vi "UI Loop - RT Target Monitoring.vi"(11 "Message Queue Reference":refnum<queue> caption="消息队列引用") -> ()   [LabVIEW 2015]
uses:
  Support VIs/Message Queue/Message Cluster.ctl
  Globals/Global - All UI Loop Stop.vi
  Support VIs/Message Queue/Message Queue.lvlib
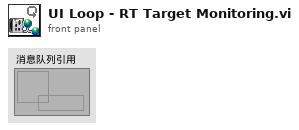
[diagram p1: front panel]
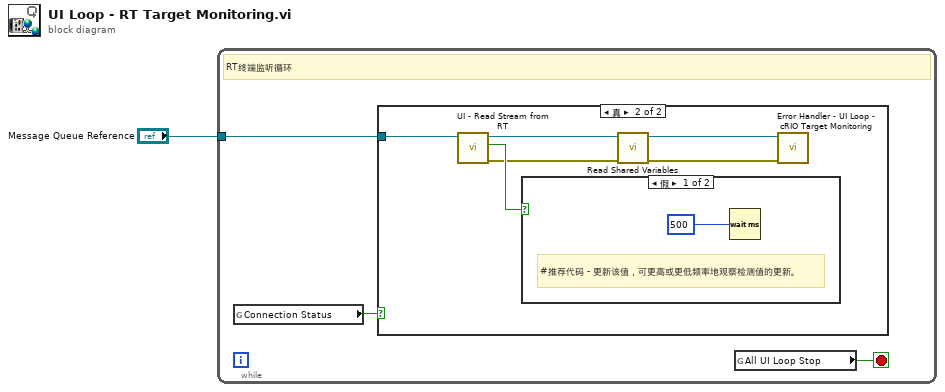
[diagram p0: block diagram]
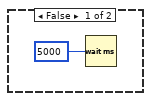
[diagram p2: hidden frame]
diagram:
  n1 = while {
    tunnel: "Message Queue Reference" -> [w3]
    stop <- w4 stop-if-true
    # "RT终端监听循环"
    n2 = global read "Global - All UI Loop Stop.vi" "Connection Status"() -> (w2:bool)
    n3 = case shown="真" w2 {
      tunnel: w3 -> [_ w11]
      frame False {
        n4 = Wait (ms)(milliseconds to wait=u32 5000 ("等待时间（毫秒）")) -> ()  [unwired: 1 out]
      }
      frame True {
        n5 = call "UI - Read Stream from RT.vi"("Message Queue"=w11) -> ("error out"=w9:errorcluster, "Message Received?"=w10:bool, "dup Message Queue"=w8:refnum<queue>)  [unwired: 8 in]
        n6 = case shown="假" w10 {
          frame False {
            # "#推荐代码 - 更新该值，可更高或更低频率地观察检测值的更新。"
            n7 = Wait (ms)(milliseconds to wait=u32 500) -> ()  [unwired: 1 out]
          }
          frame True {
            # "收到消息后，立即再次读取"
          }
        }
        n8 = call "Read Shared Variables.vi"("error in (no error)"=w9, "Message Queue"=w8) -> ("Error Out"=w7:errorcluster, "dup Message Queue"=w6:refnum<queue>)  [unwired: 7 in, 1 out]
        n9 = call "Error Handler - UI Loop - cRIO Target Monitoring.vi"("error in (no error)"=w7, "Message Queue"=w6) -> ()  [unwired: 9 in, 1 out]
      }
    }
    n10 = global read "Global - All UI Loop Stop.vi" "All UI Loop Stop"() -> (w4:bool)
  }
